vi "FindPartContact.vi"(6 "Response actuator":i8, 8 "Error In":errorcluster, 9 "Type of operation":i8, 10 "Actuator command":i32, 11 "connection ID":refnum<k5>) -> (0 "Error Out":errorcluster, 1 "Absolute distance mm":dbl, 2 "Absolute distance inch":dbl, 3 "connection ID out":refnum<k5>, 4 "Pre Part contact inch":dbl, 5 "Pre Part Contact mm":dbl)   [LabVIEW 2017]
panel:
  # "ACTUATOR SETUP : FIND PART CONTACT"
  # "Absolute distance"
  # "PrePartContact"
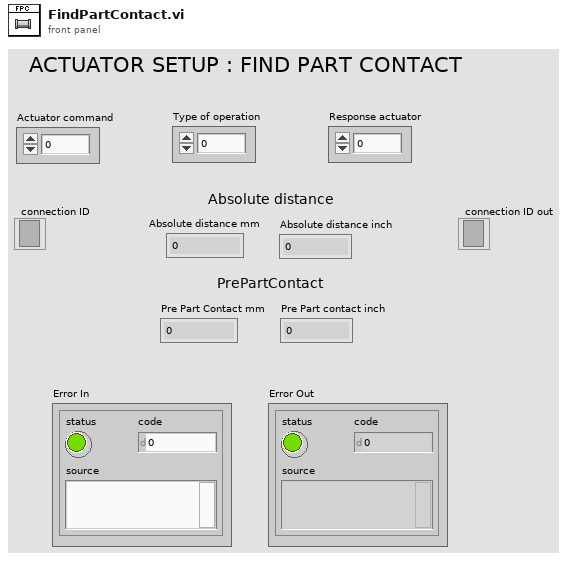
[diagram p1: front panel]
types:
  T1 = enum16{"big-endian, network order", "native, host order", "little-endian"}
  T2 = enum16{"Standard", "Buffered", "CRLF", "Immediate"}
  T3 = cluster{"Type of operation":i8, i32, "Actuator command":i32}
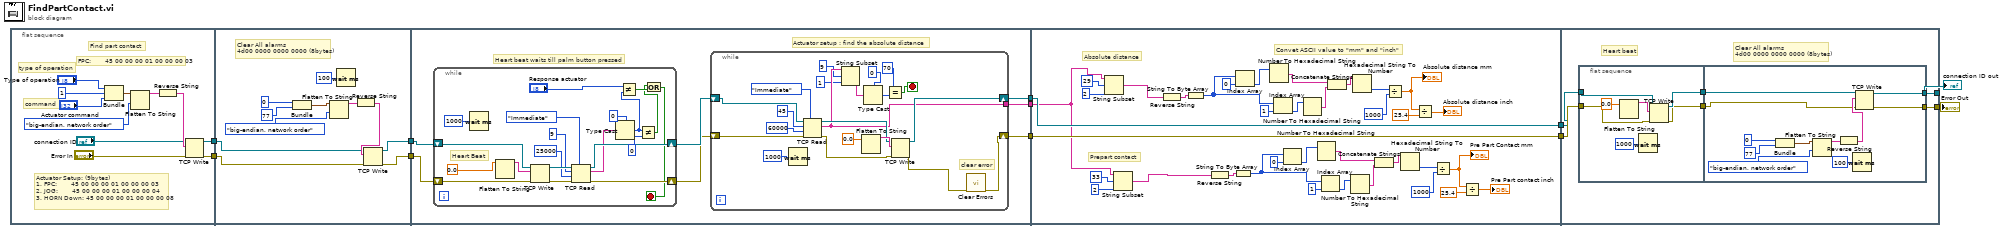
[diagram p0: block diagram]
diagram:
  n1 = flat-sequence {
    tunnel: [w20] -> w6
    tunnel: [w19] -> w4
    tunnel: w6 -> [w26]
    tunnel: [w24] -> w5
    tunnel: w4 -> [w25]
    tunnel: [w23] -> w3
    tunnel: w5 -> [w40]
    tunnel: w3 -> [w39]
    tunnel: [w38] -> w11
    tunnel: [w37] -> w10
    tunnel: [w34] -> w9
    tunnel: w11 -> [w103]
    tunnel: w10 -> [w104]
    tunnel: w9 -> [w97]
    tunnel: [w104] -> w8
    tunnel: [w103] -> w7
    tunnel: w8 -> [w124]
    tunnel: w7 -> [w123]
    tunnel: [w120] -> w2
    tunnel: [w119] -> w1
    frame #0 {
      # "type of operation"
      # "command"
      # "Actuator Setup: (9bytes)\n1. FPC:       45 00 00 00 01 00 00 00 03\n2. JOG:       45 00 00 00 01 00 00 00 04\n3. HORN Down: 45 00 00 00 01 00 00 00 08"
      # "Find part contact"
      # "FPC:       45 00 00 00 01 00 00 00 03"
      n2 = Bundle("Type of operation"="Type of operation", 1, "Actuator command"="Actuator command") -> (w17:T3)  [unwired: 1 in]
      n3 = Flatten To String(anything=w17, byte order (0:big-endian, network order)=T1."big-endian, network order") -> (data string=w22:string)  [unwired: 2 in, 2 out]
      n4 = Reverse String(1:w22) -> (0:w21:string)
      n5 = TCP Write(connection ID="connection ID", data in=w21, error in (no error)="Error In") -> (connection ID out=w20:refnum<k5>, error out=w19:errorcluster)  [unwired: 1 in, 1 out]
    }
    frame #1 {
      # "Clear All alarms\n4d00 0000 0000 0000 (8bytes)"
      n6 = Bundle(0, 77) -> (w33:cluster{i32, i32})  [unwired: 1 in]
      n7 = Flatten To String(anything=w33, byte order (0:big-endian, network order)=T1."big-endian, network order") -> (data string=w32:string)  [unwired: 2 in, 2 out]
      n8 = Wait (ms)(milliseconds to wait=u32 100) -> ()  [unwired: 1 out]
      n9 = Reverse String(1:w32) -> (0:w28:string)
      n10 = TCP Write(connection ID=w26, data in=w28, error in (no error)=w25) -> (connection ID out=w24:refnum<k5>, error out=w23:errorcluster)  [unwired: 1 in, 1 out]
    }
    frame #2 {
      # "Actuator setup : find the absolute distance"
      # "Heart beat waits till palm button pressed"
      n11 = while {
        shift-right: [w58] -> w36
        shift-left: w40 -> [w60]
        shift-right: [w57] -> w35
        shift-left: w39 -> [w59]
        stop <- w45 stop-if-true
        # "Heart Beat"
        n12 = Wait (ms)(milliseconds to wait=u32 1000) -> ()  [unwired: 1 out]
        n13 = Flatten To String(anything=0.0) -> (data string=w55:string)  [unwired: 3 in, 2 out]
        n14 = TCP Write(connection ID=w60, data in=w55, error in (no error)=w59) -> (connection ID out=w54:refnum<k5>, error out=w53:errorcluster)  [unwired: 1 in, 1 out]
        n15 = TCP Read(connection ID=w54, bytes to read=9, error in (no error)=w53, 7:T2."Immediate" ("mode (standard)"), 9:25000 ("timeout ms (25000)")) -> (connection ID out=w58:refnum<k5>, data out=w48:string, error out=w57:errorcluster)
        n16 = Type Cast(type=u8 0, x=w48) -> (*(type *) &x=w42:u8)
        n17 = Not Equal?(x="Response actuator", y=w42) -> (x != y?=w44:bool)
        n18 = Not Equal?(x=w42, y=u8 0) -> (x != y?=w43:bool)
        n19 = Or(x=w43, y=w44) -> (x .or. y?=w45:bool)
      }
      n20 = while {
        tunnel: [w67] -> w34
        shift-right: [w69] -> w38
        shift-left: w36 -> [w81]
        shift-right: [w68] -> w37
        shift-left: w35 -> [w80]
        stop <- w75 stop-if-true
        # "clear error"
        n21 = Wait (ms)(milliseconds to wait=u32 1000) -> ()  [unwired: 1 out]
        n22 = TCP Read(connection ID=w81, bytes to read=45, error in (no error)=w80, 7:T2."Immediate" ("mode (standard)"), 9:60000 ("timeout ms (25000)")) -> (connection ID out=w72:refnum<k5>, data out=w67:string, error out=w71:errorcluster)
        n23 = String Subset(string=w67, offset (0)=9, length (rest)=1 ("length (rest)")) -> (substring=w62:string)
        n24 = Flatten To String(anything=0.0) -> (data string=w73:string)  [unwired: 3 in, 2 out]
        n25 = Type Cast(type=u8 0, x=w62) -> (*(type *) &x=w64:u8)
        n26 = Equal?(x=u8 70, y=w64) -> (x = y?=w75:bool)
        n27 = TCP Write(connection ID=w72, data in=w73, error in (no error)=w71) -> (connection ID out=w69:refnum<k5>, error out=w70:errorcluster)  [unwired: 1 in, 1 out]
        n28 = call <vilib>:"Clear Errors.vi"("error in (no error)"=w70) -> ("error out"=w68:errorcluster)  [unwired: 5 in, 1 out]
      }
    }
    frame #3 {
      # "Convet ASCII value to \"mm\" and \"inch\""
      # "Prepart contact"
      # "Absolute distance"
      n29 = String Subset(string=w97, offset (0)=29, length (rest)=2 ("length (rest)")) -> (substring=w116:string)
      n30 = String Subset(string=w97, offset (0)=33, length (rest)=2 ("length (rest)")) -> (substring=w82:string)
      n31 = Reverse String(1:w116) -> (0:w115:string)
      n32 = String To Byte Array(string=w115) -> (unsigned byte array=w110:u8[])
      n33 = Reverse String(1:w82) -> (0:w83:string)
      n34 = String To Byte Array(string=w83) -> (unsigned byte array=w88:u8[])
      n35 = Index Array(array=w110, index=0) -> (element=w113:u8)
      n36 = Number To Hexadecimal String(2:w113) -> (0:w108:string)  [unwired: 1 in]
      n37 = Index Array(array=w110, index=1) -> (element=w112:u8)
      n38 = Index Array(array=w88, index=0) -> (element=w85:u8)
      n39 = Number To Hexadecimal String(2:w112) -> (0:w109:string)  [unwired: 1 in]
      n40 = Number To Hexadecimal String(2:w85) -> (0:w90:string)  [unwired: 1 in]
      n41 = Index Array(array=w88, index=1) -> (element=w86:u8)
      n42 = Concatenate Strings(w108, w109) -> (w107:string)
      n43 = Number To Hexadecimal String(2:w86) -> (0:w89:string)  [unwired: 1 in]
      n44 = Hexadecimal String To Number(string=w107) -> (number=w106:u32)  [unwired: 2 in, 1 out]
      n45 = Concatenate Strings(w90, w89) -> (w91:string)
      n46 = Divide(x=w106, y=1000) -> (x/y=w102:dbl)
      "Absolute distance mm" <- w102
      n47 = Hexadecimal String To Number(string=w91) -> (number=w92:u32)  [unwired: 2 in, 1 out]
      n48 = Divide(x=w102, y=25.4) -> (x/y=→"Absolute distance inch":dbl)
      n49 = Divide(x=w92, y=1000) -> (x/y=w94:dbl)
      "Pre Part Contact mm" <- w94
      n50 = Divide(x=w94, y=25.4) -> (x/y=→"Pre Part contact inch":dbl)
    }
    frame #4 {
      # "Clear All alarms\n4d00 0000 0000 0000 (8bytes)"
      # "Heart beat"
      n51 = flat-sequence {
        tunnel: w124 -> [w126]
        tunnel: w123 -> [w128]
        tunnel: [w127] -> w122
        tunnel: [w125] -> w121
        tunnel: w122 -> [w136]
        tunnel: w121 -> [w135]
        tunnel: [w133] -> w120
        tunnel: [w132] -> w119
        frame #0 {
          n52 = Flatten To String(anything=0.0) -> (data string=w129:string)  [unwired: 3 in, 2 out]
          n53 = Wait (ms)(milliseconds to wait=u32 1000) -> ()  [unwired: 1 out]
          n54 = TCP Write(connection ID=w128, data in=w129, error in (no error)=w126) -> (connection ID out=w127:refnum<k5>, error out=w125:errorcluster)  [unwired: 1 in, 1 out]
        }
        frame #1 {
          n55 = Bundle(0, 77) -> (w142:cluster{i32, i32})  [unwired: 1 in]
          n56 = Flatten To String(anything=w142, byte order (0:big-endian, network order)=T1."big-endian, network order") -> (data string=w141:string)  [unwired: 2 in, 2 out]
          n57 = Reverse String(1:w141) -> (0:w137:string)
          n58 = Wait (ms)(milliseconds to wait=u32 100) -> ()  [unwired: 1 out]
          n59 = TCP Write(connection ID=w136, data in=w137, error in (no error)=w135) -> (connection ID out=w132:refnum<k5>, error out=w133:errorcluster)  [unwired: 1 in, 1 out]
        }
      }
    }
  }
  "Error Out" <- w2
  "connection ID out" <- w1
